vi "Get Selftuning.vi"(8 "error in":errorcluster, 11 "VISA resource name in":refnum<visa-resource-name>) -> (0 "error out":errorcluster, 1 "Selftuning (out)":enum16{"OFF", "ONCE", "ALWAYS"}(ring), 3 "VISA resource name out":refnum<visa-resource-name>)   [LabVIEW 2015, in "JULABO DeviceDriver.lvlib"]
doc: "This VI returns the status of the optimization process for internal and external control parameters.\n\n<B>Meaning:</B>\n<B>off - no selftuning</B>\nThe control parameters ascertained during the last identification are\nused for control purposes.\n<B>once - single selftuning</B>\nThe instrument performs a single selftuning of the controlled system after each start with the key or after receiving a start command via the interface.\n<B>always - continual selftuning</B>\nThe instrument performs a selftuning of the controlled system whenever a new setpoint is to be reached. Use this setting only when the temperature application system changes permanently."
uses:
  JULABO DeviceDriver.lvlib
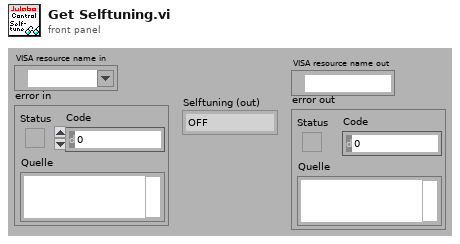
[diagram p1: front panel]
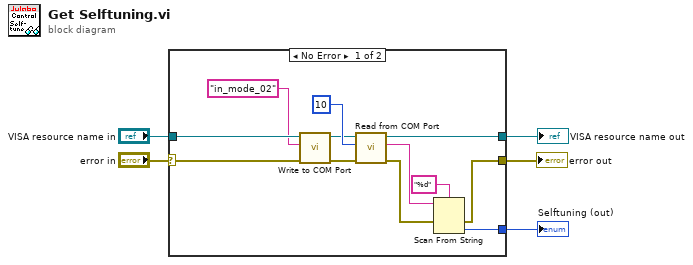
[diagram p0: block diagram]
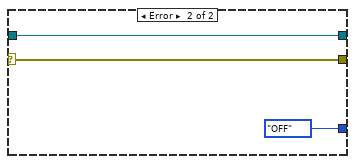
[diagram p2: hidden frame]
diagram:
  n1 = case shown="No Error" "error in" {
    selector: "error in" -> [w14 w19]
    tunnel: [w17 w20] -> w5
    tunnel: "VISA resource name in" -> [w16 w20]
    tunnel: [w15 w19] -> w3
    tunnel: [w6 enum16{"OFF", "ONCE", "ALWAYS"}."OFF" ("Selftuning (out)")] -> w1
    frame No Error {
      n2 = call "Write to COM Port.vi"("error in"=w14, "Command (input)"="in_mode_02" ("Schreibpuffer"), "VISA resource name in"=w16) -> ("error out"=w9:errorcluster, "VISA resource name out"=w10:refnum<visa-resource-name>)  [unwired: 7 in]
      n3 = call "Read from COM Port.vi"("error in"=w9, "Byte to Read (-1:All)"=u32 10 ("Anzahl der Byte"), "VISA resource name in"=w10) -> ("error out"=w7:errorcluster, "String (output)"=w12:string, "VISA resource name out"=w17:refnum<visa-resource-name>)  [unwired: 5 in, 1 out]
      n4 = Scan From String(format string="%d" ("Format-String"), input string=w12, error in=w7) -> (error out=w15:errorcluster, output 1=w6:i32)  [unwired: 2 in, 2 out]
    }
    frame Error {
    }
  }
  "VISA resource name out" <- w5
  "error out" <- w3
  "Selftuning (out)" <- w1
